vi "OE1311&OE1351_RS232_Query Data.vi"(0 "VISA resource name":refnum<visa-resource-name>, 11 "Error in (no error)":errorcluster caption="error out（no error）") -> (4 "VISA resource  out":refnum<visa-resource-name>, 6 "Data Array":dbl[](array[numeric]), 8 "Parameter Values":T1, 10 "Output String":string, 15 "Error out":errorcluster caption="error out")   [LabVIEW 2011]
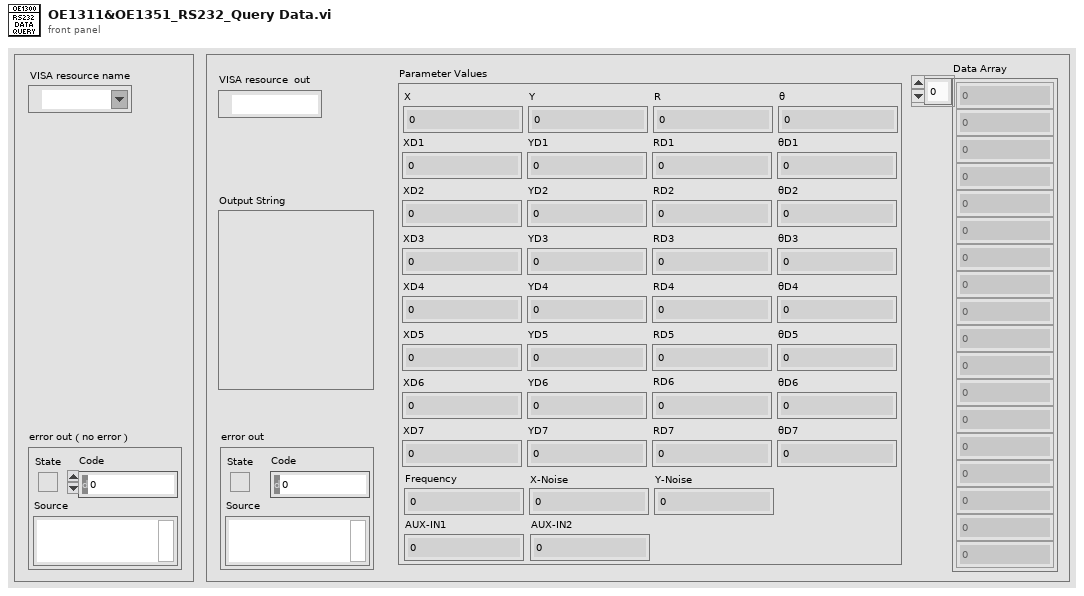
[diagram p1: front panel]
types:
  T1 = cluster{"X":dbl, "Y":dbl, "R":dbl, "θ":dbl, "XD1":dbl, "YD1":dbl, "RD1":dbl, "θD1":dbl, "XD2":dbl, "YD2":dbl, "RD2":dbl, "θD2":dbl, "XD3":dbl, "YD3":dbl, "RD3":dbl, "θD3":dbl, "XD4":dbl, "YD4":dbl, "RD4":dbl, "θD4":dbl, "XD5":dbl, "YD5":dbl, "RD5":dbl, "θD5":dbl, "XD6":dbl, "YD6":dbl, "RD6":dbl, "θD6":dbl, "XD7":dbl, "YD7":dbl, "RD7":dbl, "θD7":dbl, "X-Noise":dbl, "Y-Noise":dbl, "Frequency":dbl, "AUX-IN1":dbl, "AUX-IN2":dbl}
  T2 = enum16{"ISRC", "IGND", "ICPL", "ILIN", "PHAS", "FMOD", "RSLP", "FREQ", "SWPT", "SLLM", "SULM", "SSLL", "SSLG", "STLM", "SWRM", "IRNG", "SENS", "RMOD", "OFLT", "OFSL", "SYNC", "DMOD", "HARM", "DARB", "SWVT", "SLVL", "SVLL", "SVUL", "SVSL", "SVSG", "SVTM", "SVRM", "RALL", "SNAP", "OUTP", "OAUX", "COUT", "CAUX", "COFP", "CEXP", "FPOP", "OEXP", "*IDN", "*RST", "OVLD", "INOV", "GNOV", "*PLL", "SSET", "RSET", "AGAN", "APHS", "ARSV", "ASCL", "EQCD", "EQCS", "SPED", "SRAT", "SLEN", "SSLE", "STRG", "SPRM", "STRD", "PAUS", "REST", "SPTS", "TRCA", "TEMP", "RSTU", "IHNZ", "DEQU", "SADD", "ARNG", "CSPE", "ISRCD", "IGNDD", "ICPLD", "ILIND", "PHASD", "FMODD", "RSLPD", "FREQD", "SWPTD", "SLLMD", "SULMD", "SSLLD", "SSLGD", "STLMD", "SWRMD", "SENSD", "RMODD", "OFLTD", "OFSLD", "SYNCD", "HARMD", "EQCDD", "EQCSD", "SNAPD", "OUTPD", "SWVTD", "SLVLD", "SVLLD", "SVULD", "SVSLD", "SVSGD", "SVTMD", "SVRMD", "SVDCD", "ARSVD", "AGAND", "APHSD", "ASCLD", "FPOPD", "CAUXD", "OEXPD", "SPEDD", "SRATD", "SLEND", "SSLED", "STRGD", "SPRMD", "STRDD", "PAUSD", "RESTD", "SPTSD", "TRCAD", "*IDND", "*RSTD", "INOVD", "GNOVD", "*PLLD", "SSETD", "RSETD", "RALLD"}
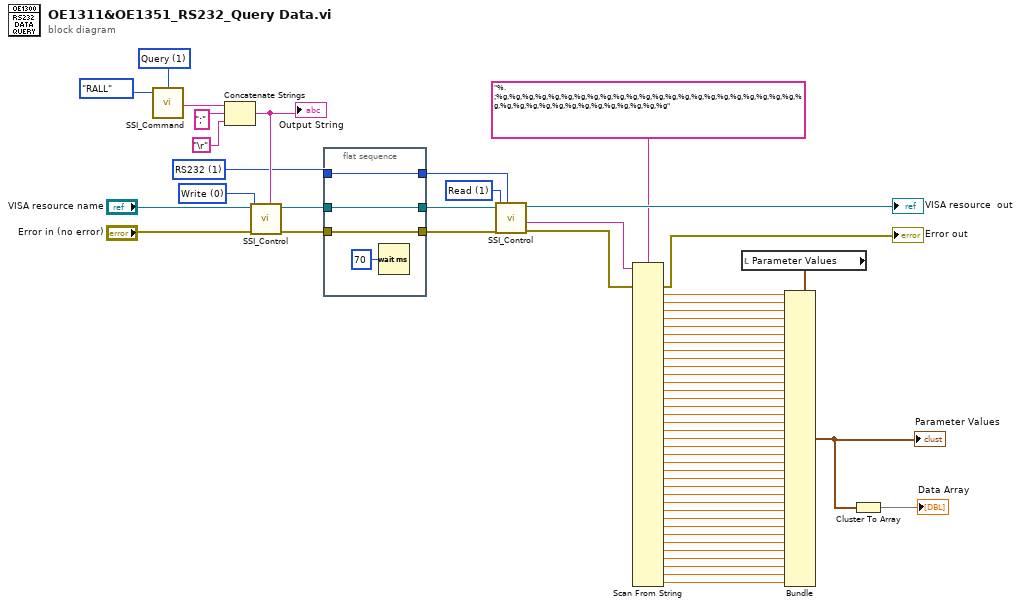
[diagram p0: block diagram]
diagram:
  w3 = u16 1 items=["USB", "RS232", "GPIB", "Ethernet"] ("Remote Mode")
  w8 = u16 1 items=["Set", "Query"] ("Opera")
  w53 = u16 1 items=["Write", "Read"] ("Control")
  w58 = u16 0 items=["Write", "Read"] ("Control")
  n1 = call "SSI_Command.vi"("Opera"=w8, "Command Type"=T2."RALL") -> ("Output string"=w7:string)  [unwired: 2 in]
  n2 = Concatenate Strings(w7, ";" ("字符串"), "\r") -> (w11:string)
  "Output String" <- w11
  n3 = call "SSI_Control.vi"("Write Buffer"=w11, "Error in (no error)"="Error in (no error)", "Control"=w58, "VISA resource name"="VISA resource name") -> ("Error out"=w56:errorcluster, "VISA resource  out"=w57:refnum<visa-resource-name>)  [unwired: 4 in, 2 out]
  n4 = flat-sequence {
    tunnel: w57 -> [w65]
    tunnel: w56 -> [w64]
    tunnel: [w65] -> w55
    tunnel: [w64] -> w54
    tunnel: [w62] -> w4
    tunnel: w3 -> [w62]
    frame #0 {
      n5 = Wait (ms)(milliseconds to wait=u32 70 ("等待时间（毫秒）")) -> ()  [unwired: 1 out]
    }
  }
  n6 = call "SSI_Control.vi"("Remote Mode"=w4, "Error in (no error)"=w54, "Control"=w53, "VISA resource name"=w55) -> ("Error out"=w52:errorcluster, "Read Buffer"=w5:string, "VISA resource  out"=→"VISA resource  out":refnum<visa-resource-name>)  [unwired: 4 in, 1 out]
  n7 = Scan From String(format string="%.;%g,%g,%g,%g,%g,%g,%g,%g,%g,%g,%g,%g,%g,%g,%g,%g,%g,%g,%g,%g,%g,%g,%g,%g,%g,%g,%g,%g,%g,%g,%g,%g,%g,%g,%g,%g,%g" ("格式字符串"), input string=w5, error in=w52) -> (error out=→"Error out":errorcluster, output 1=w50:dbl, output 2=w49:dbl, output 3=w48:dbl, output 4=w47:dbl, output 5=w46:dbl, output 6=w44:dbl, output 7=w43:dbl, output 8=w42:dbl, output 9=w41:dbl, output 10=w40:dbl, output 11=w39:dbl, output 12=w35:dbl, output 13=w34:dbl, output 14=w33:dbl, output 15=w32:dbl, output 16=w31:dbl, output 17=w30:dbl, output 18=w29:dbl, output 19=w36:dbl, output 20=w37:dbl, output 21=w38:dbl, output 22=w45:dbl, output 23=w28:dbl, output 24=w26:dbl, output 25=w25:dbl, output 26=w24:dbl, output 27=w23:dbl, output 28=w22:dbl, output 29=w21:dbl, output 30=w20:dbl, output 31=w19:dbl, output 32=w18:dbl, output 33=w17:dbl, output 34=w16:dbl, output 35=w15:dbl, output 36=w14:dbl, output 37=w13:dbl)  [unwired: 38 in, 2 out]
  n8 = local read "Parameter Values"() -> (w12:T1)
  n9 = Bundle(cluster=w12, "X"=w50, "Y"=w49, "R"=w48, "θ"=w47, "XD1"=w46, "YD1"=w44, "RD1"=w43, "θD1"=w42, "XD2"=w41, "YD2"=w40, "RD2"=w39, "θD2"=w35, "XD3"=w34, "YD3"=w33, "RD3"=w32, "θD3"=w31, "XD4"=w30, "YD4"=w29, "RD4"=w36, "θD4"=w37, "XD5"=w38, "YD5"=w45, "RD5"=w28, "θD5"=w26, "XD6"=w25, "YD6"=w24, "RD6"=w23, "θD6"=w22, "XD7"=w21, "YD7"=w20, "RD7"=w19, "θD7"=w18, "X-Noise"=w17, "Y-Noise"=w16, "Frequency"=w15, "AUX-IN1"=w14, "AUX-IN2"=w13) -> (w2:T1)
  "Parameter Values" <- w2
  n10 = Cluster To Array(cluster=w2) -> (array=→"Data Array":dbl[])
